vi "Dashboard Main.vi"() -> ()   [LabVIEW 2020]
uses:
  <vilib>/event_ctls.llb/eventvkey.ctl
  <vilib>/Rock Robotics/WPI/ThirdParty/JAS_Junk/TrajLib/TypeDef/TRANSLATION2D.ctl
  d5e2e769-f078-4149-bfe1-3f7844503895.vi
  <vilib>/Rock Robotics/WPI/ThirdParty/JAS_Junk/TrajLib/Conv_Radians_Deg.vi
  <vilib>/Rock Robotics/WPI/ThirdParty/JAS_Junk/TrajLib/Conv_Deg_Radians.vi
  <vilib>/Rock Robotics/WPI/ThirdParty/JAS_Junk/TrajLib/Rotation2d_CreateAngle.vi
  <vilib>/Rock Robotics/WPI/ThirdParty/JAS_Junk/TrajLib/Translation2d_Create.vi
  <vilib>/Rock Robotics/WPI/ThirdParty/JAS_Junk/TrajLib/VI/Util_GetTime_U32.vi
  <vilib>/Rock Robotics/Network Tables/NT Read Numeric Array.vi
  <vilib>/Rock Robotics/WPI/ThirdParty/JAS_Junk/TrajLib/VI/Util_GetTime_U64.vi
  <vilib>/Rock Robotics/WPI/Dashboard/WPI_DashboardLogging Global.vi
  <vilib>/picture/picture.llb/Draw True-Color Pixmap.vi
  <vilib>/Rock Robotics/WPI/ThirdParty/JAS_Junk/TrajLib/Trajectory_Library.lvlib
  <vilib>/vision/NI_Vision_Development_Module.lvlib
panel:
  in  "Camera Settings Right":T1={"Frame Rate"=30, "Compression"=30, "Size"=1, "DB Camera Config"=FALSE} {"Frame Rate" scale=1.0..30.0; "Compression" scale=100.0..-1.0; "Size" items=["640x480", "320x240", "160x120"]}
  in  "Camera Name Right":string(combo)="No Camera Selection"
  out "Camera Perf":string
  in  "Camera Settings":T1={"Frame Rate"=30, "Compression"=30, "Size"=1, "DB Camera Config"=FALSE} {"Frame Rate" scale=1.0..30.0; "Compression" scale=100.0..-1.0; "Size" items=["640x480", "320x240", "160x120"]}
  in  "TCP":refnum<k5>
  in  "Rec Mode":enum32{"Stop", "Record", "Playback"}(radio)
  out "Robot IP":string
  out "Image Message":string="Timeout in Camera Communications"
  in  "Dashboard Tab":T2(tab)
  in  "Select Auto":string(combo)="Select Autonomous ..."
  out "NT Connection":bool
  out "MotorChart R":cluster{"Numeric":dbl, "Numeric":dbl}(graph)
  out "MotorChart L":cluster{"Numeric":dbl, "Numeric":dbl}(graph)
  out "MotorSliders R":cluster{"MotorSlide1":dbl, "MotorSlide2":dbl} {"MotorSlide2" scale=-1.0..1.0 scale format="%#_2e"; "MotorSlide1" scale=-1.0..1.0 scale format="%#_2e"}
  out "MotorSliders L":cluster{"MotorSlide1":dbl, "MotorSlide2":dbl} {"MotorSlide2" scale=-1.0..1.0 scale format="%#_2e"; "MotorSlide1" scale=-1.0..1.0 scale format="%#_2e"}
  out "Gyro":dbl(knob) scale=0.0..360.0
  out "JS1 Z":dbl(slide) scale=-1.0..1.0 scale format="%#_2e"
  out "JS1 Graph":cluster{"X":dbl, "Y":dbl}[](graph)
  out "JS1 Buttons":T3
  out "JS2 Z":dbl(slide) scale=-1.0..1.0 scale format="%#_2e"
  out "JS2 Graph":cluster{"X":dbl, "Y":dbl}[](graph)
  out "JS2 Buttons":T3
  out "Mode":T4(ring)=enum."Auto Disabled"
  out "Right Camera Perf":cluster{"Bandwidth (Mbps)":dbl, "FPS":dbl}
  out "Camera Image Right":T5(plugin-control)
  in  "DB/String 9":string
  in  "DB/String 8":string
  in  "DB/String 7":string
  in  "DB/String 6":string
  in  "DB/String 5":string
  in  "DB/String 4":string
  in  "DB/String 3":string
  in  "DB/String 2":string
  in  "DB/String 1":string
  in  "DB/String 0":string
  in  "DB/Slider 0":dbl(slide) scale=0.0..5.0
  in  "DB/Slider 1":dbl(slide) scale=0.0..5.0
  in  "DB/Slider 2":dbl(slide) scale=0.0..5.0
  in  "DB/Slider 3":dbl(slide) scale=0.0..5.0
  out "DB/LED 3":bool
  out "DB/LED 2":bool
  out "DB/LED 1":bool
  out "DB/LED 0":bool
  in  "DB/Button 3":bool
  in  "DB/Button 2":bool
  in  "DB/Button 1":bool
  in  "DB/Button 0":bool caption="New Name"
  out "PID Chart":cluster{"X":dbl[], "Y":dbl[]}[](graph)
  out "LF PIDF":dbl[](array[numeric])
  out "c(t)":dbl
  out "time":dbl
  in  "PID Ctrl":dbl[](array[numeric])=[0.7, 0.0, 0.0]
  out "r(t)":dbl
  in  "PV (NT Name)":string="ActualPoseX"
  in  "SP (NT Name)":string="SamplePoseX"
  out "Field":cluster{dbl[], dbl[]}[](graph)
  out "Current Time":dbl
  in  "Test Slider":dbl(slide) scale=0.0..100.0 scale format="%#_3g"
  in  "On/Off":bool caption="Solenoid"
  in  "Test Name":u16(ring) items=["Select the test to run..."]
  in  "Test Tree":string(tree)
  in  "Motor":cluster{"Value":dbl, "Enable":bool} {"Value" scale=-1.0..1.0 scale format="%#_3g"}
  out "Progress":T6 {"Test Progress" scale=0.0..100.0}
  in  "Rev/Fwd":cluster{"Forward":bool, "Reverse":bool}
  in  "Test Ring":u16(ring) items=["Monochrome", "Color"]
  in  "CheckList":i32(listbox)
  out "Tree":string(tree)
  out "Camera Image":T5(plugin-control)
  out "Background":bool
  in  "Camera Name":string(combo)="No Camera Selection"
  # "HW"
  # "HW"
  # "Joysticks"
  # "Drive Motors"
  # "Front"
  # "Right"
  # "Left"
  # "Back"
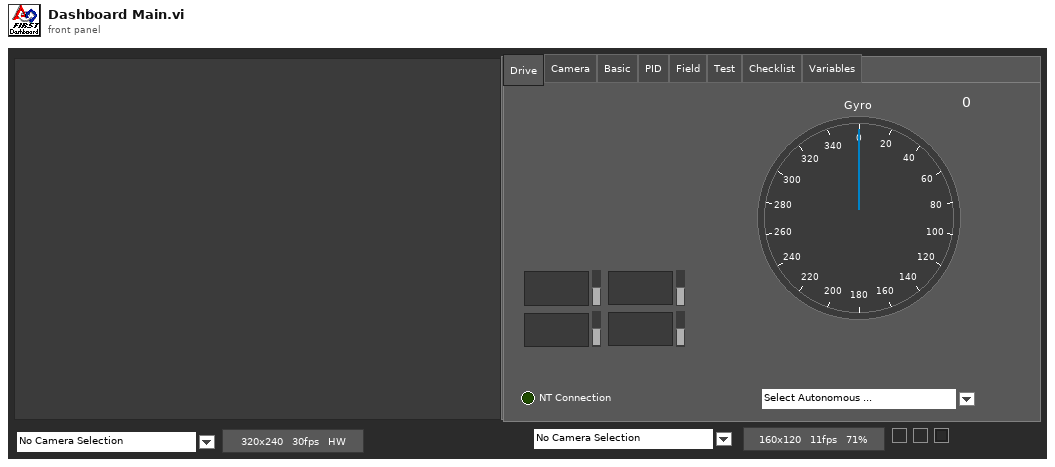
[diagram p1: front panel]
types:
  T1 = cluster{"Frame Rate":i32, "Compression":i32, "Size":u16, "DB Camera Config":bool}
  T2 = enum32{"Drive", "Camera", "Basic", "PID", "Field", "Test", "Checklist", "Variables"}
  T3 = cluster{bool, bool, bool, bool, bool, bool, bool, bool, bool, bool, bool, bool}
  T4 = enum8{"Tele-Op Disabled", "Tele-Op Enabled", "Auto Disabled", "Auto Enabled", "Test Disabled", "Test Enabled", "Disconnected", "No Code", "E-Stop"}
  T5 = typedef "IMAQ Image.ctl" = refnum<image>
  T6 = cluster{"Test Progress":u8, "Test Progress Text":string}
  T7 = typedef "Image Type" = u32
  T8 = cluster{"Save Path":path, "Interval (s)":dbl, "Keep":i32}
  T9 = enum32{"Drive", "Camera", "Basic", "Custom", "Test", "Commands", "Checklist", "Variables"}
  T10 = cluster{"Error Strings":string, "Disable Counts":cluster{u16, u16}, "Rail Faults":cluster{u16, u16, u16}, "Robot IP":string, "DB Mode":u8, "Event Info":cluster{"Name":string, "Type":u8, "Number":u16, "Replay":u8}}
  T11 = cluster{"Storage":cluster{"Disk Free":u64, "RAM Block":u32, "RAM free":u32}, "CPU Utilization":cluster{"CPU % ISR":sgl, "CPU % Time Crit":sgl, "CPU % Timed Str":sgl, "CPU % High":sgl, "CPU % Above":sgl, "CPU % Normal":sgl, "CPU % Low":sgl}, "CAN":cluster{"% Bus Utilization":sgl, "Bus Off Cnt":u32, "TX_FIFO Full Cnt":u32, "Receive Error Cnt":u8, "Transmit Error Cnt":u8}, "HID":cluster{"HID Outputs":u32, "Rumble Low":u16, "Rumble High":u16}[]}
  T12 = cluster{"Status bits":cluster{"Test Mode":bool, "Autonomous":bool, "Enabled":bool, "Code Start":bool, "Brownout":bool, "Reserved 2":bool, "Reserved 3":bool, "E-Stop":bool}, "Code Trace":cluster{"Disabled":bool, "TeleOp":bool, "Auto":bool, "Test":bool}, "Controller Type":enum16{"unknown", "cRIO", "roboRio"}, "Code?":enum16{"unknown", "noCode", "code"}, "Battery V":dbl}
  T13 = cluster{"Control Bits":cluster{"TestMode":bool, "Autonomous":bool, "Enabled":bool, "FMS Present":bool, bool, bool, bool, "E-Stop":bool}, "Team Station ":u8, "Countdown":sgl, "Joystick Values":cluster{"Axes":dbl[], "Buttons":bool[], "POVs":i16[]}[]}
  T14 = typedef "Trajectory_Library.lvlib/TRANSLATION2D.ctl" = cluster{"X":dbl, "Y":dbl}
  T15 = cluster{"Axes":dbl[], "Buttons":bool[], "POVs":i16[]}[]
  T16 = cluster{"Axes":dbl[], "Buttons":bool[], "POVs":i16[]}
  T17 = cluster{"Buttons[0]":bool, "Buttons[1]":bool, "Buttons[2]":bool, "Buttons[3]":bool, "Buttons[4]":bool, "Buttons[5]":bool, "Buttons[6]":bool, "Buttons[7]":bool, "Buttons[8]":bool, "Buttons[9]":bool, "Buttons[10]":bool, "Buttons[11]":bool}
  T18 = typedef "Trajectory_Library.lvlib/ROTATION2D.ctl" = cluster{"VALUE":dbl, "COS":dbl, "SIN":dbl}
  T19 = cluster{"Camera Image":refnum<vi>, "Dashboard Tab":refnum<vi>, "Background":refnum<vi>, "Rec Mode":refnum<vi>, "Test Slider":refnum<vi>, "On/Off ":refnum<vi>, "Test Ring":refnum<vi>, "Rev/Fwd":refnum<vi>, "Test Name":refnum<vi>, "Motor":refnum<vi>, "Progress":refnum<vi>, "CheckList":refnum<vi>, "Tree":refnum<vi>, "Test Tree":refnum<vi>, "Camera Settings":refnum<vi>, "Camera Name":refnum<vi>, "Camera Perf":refnum<vi>, "Camera Settings Right":refnum<vi>, "Camera Name Right":refnum<vi>, "Camera Image Right":refnum<vi>}
  T20 = cluster{"Global Rectangle":i32[], "Contours":cluster{"Contour Type":u32, "ROI Type":u32, "Points":i32[]}[]}
  T21 = cluster{"Camera Name":string, string, "Saved DB Images Info":cluster{"Save Path":path, "Interval (s)":dbl, "Keep":i32}}
  T22 = cluster{"Camera Name Right":string, string, "Saved DB Images Info":cluster{"Save Path":path, "Interval (s)":dbl, "Keep":i32}}
  T23 = cluster{"Operation":enum16{"Update", "Clear"}, "Color Box":u32}[]
  T24 = typedef "eventvkey.ctl" = enum16{"ASCII", "Enter", "Return", "Shift", "Ctrl", "Alt", "Cmd", "Opt", "Caps", "NumLock", "Clear", "Break", "Up", "Down", "Left", "Right", "Insert", "Delete", "Home", "End", "PageUp", "PageDown", "Escape", "Help", "Pause", "ScrollLock", "F1", "F2", "F3", "F4", "F5", "F6", "F7", "F8", "F9", "F10", "F11", "F12", "F13", "F14", "F15", "F16", "F17", "F18", "F19", "F20", "F21", "F22", "F23", "F24", "Play", "VolumeUp", "VolumeDown", "Mute", "Two Byte Char"}
  T25 = cluster{"Image Size":bool, "Image Type":bool, "Pixel Value":bool, "ROI Information":bool, "Zoom Factor":bool}
  T26 = cluster{"Operation":enum16{"Update", "Clear"}, "Color Box":u32}
  T27 = cluster{"Shift":bool, "Ctrl":bool, "Alt":bool, "Cmd":bool, "Opt":bool}
  T28 = typedef "imagedata.ctl" = cluster{"image type":i32, "image depth":i32, "image":u8[], "mask":u8[], "colors":u32[], "Rectangle":cluster{"left":i16, "top":i16, "right":i16, "bottom":i16}}
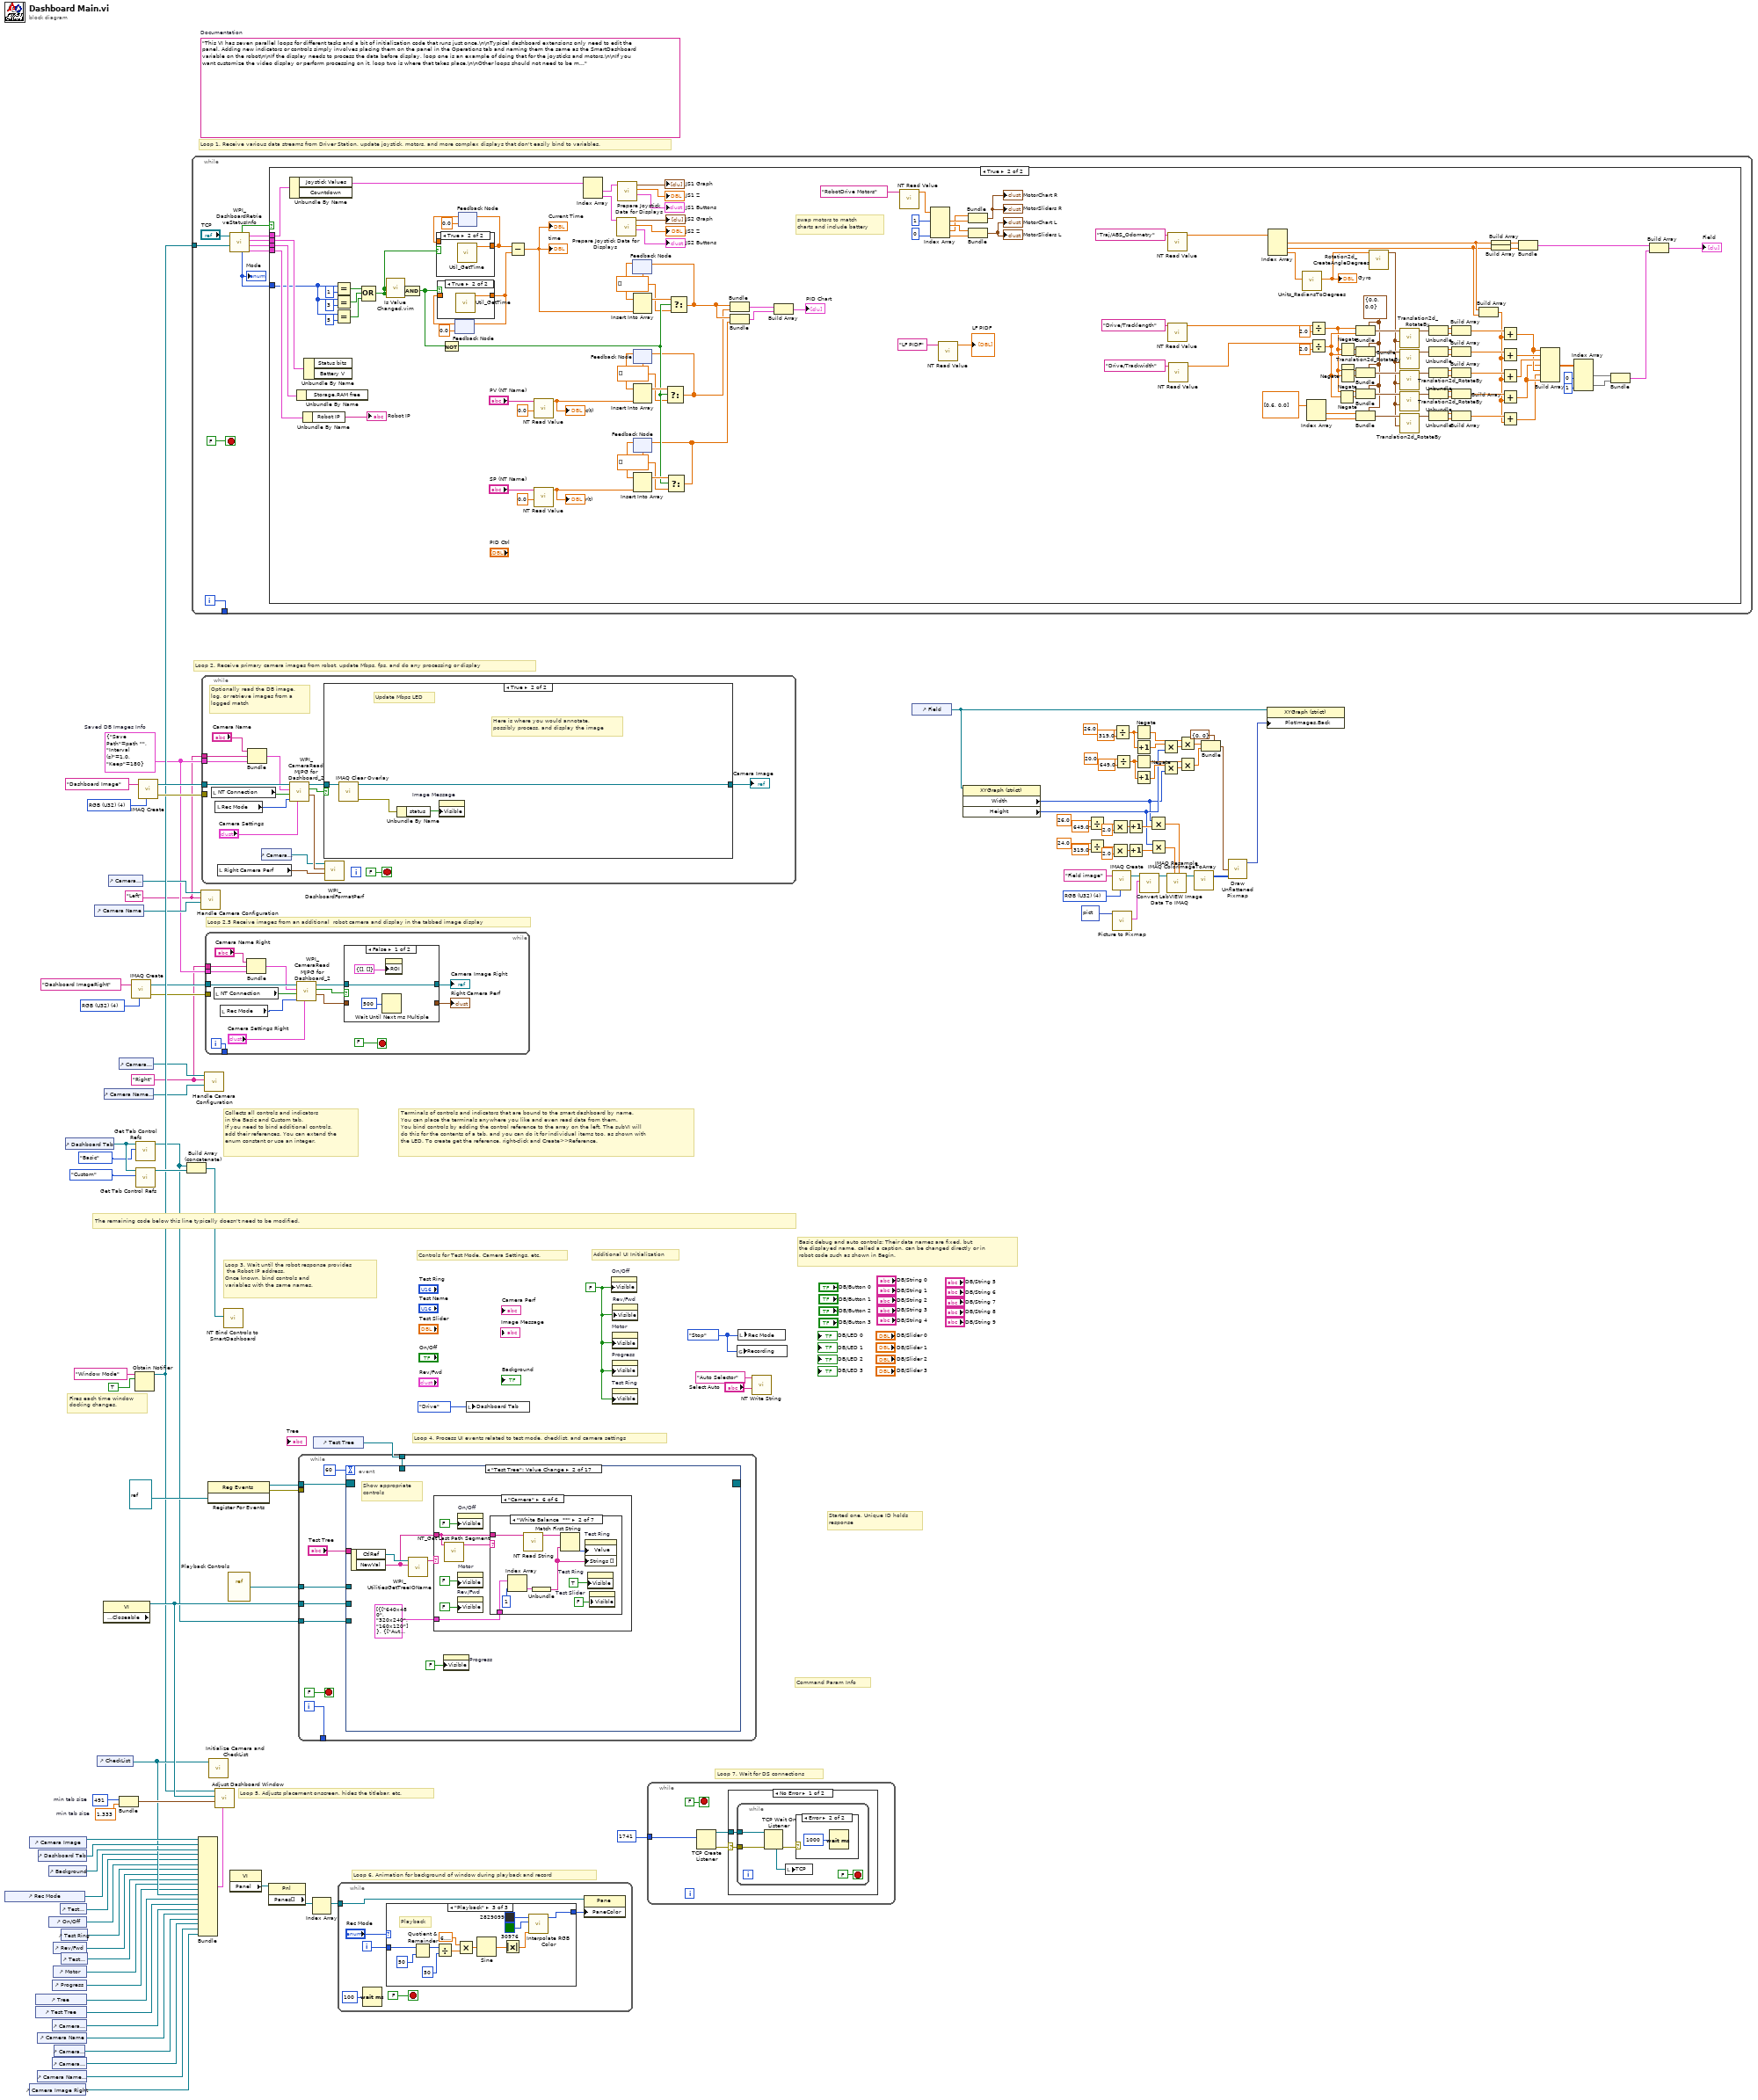
[diagram p0: block diagram]
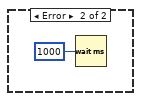
[diagram p4: hidden frame]
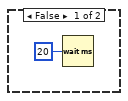
[diagram p5: hidden frame]
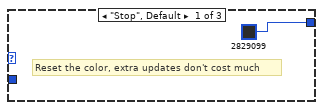
[diagram p8: hidden frame]
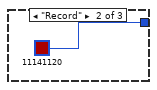
[diagram p9: hidden frame]
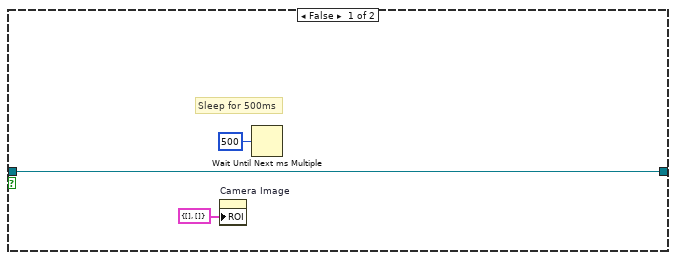
[diagram p10: hidden frame]
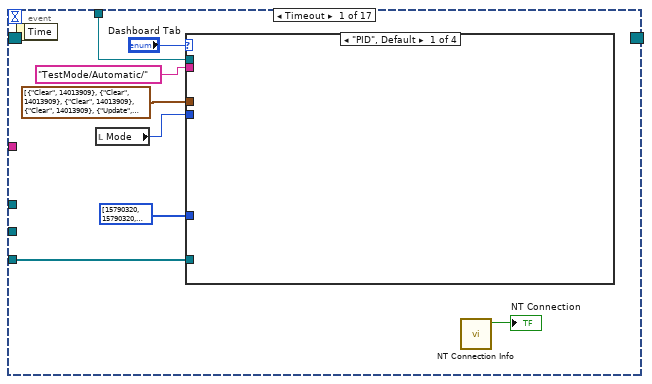
[diagram p11: hidden frame]
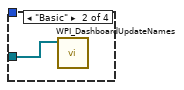
[diagram p12: hidden frame]
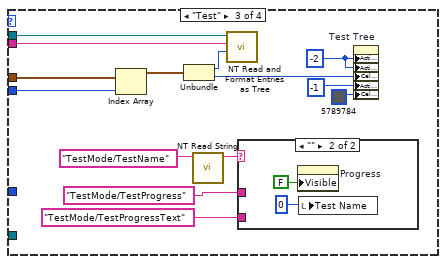
[diagram p13: hidden frame]
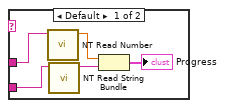
[diagram p14: hidden frame]
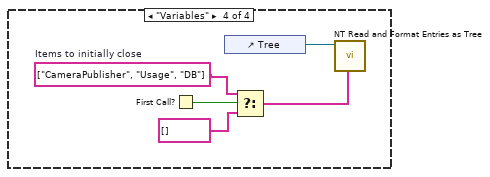
[diagram p15: hidden frame]
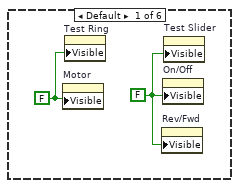
[diagram p16: hidden frame]
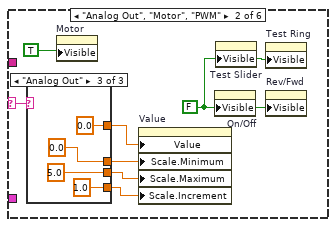
[diagram p17: hidden frame]
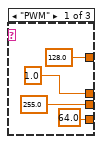
[diagram p18: hidden frame]
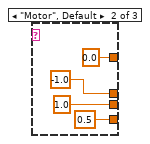
[diagram p19: hidden frame]
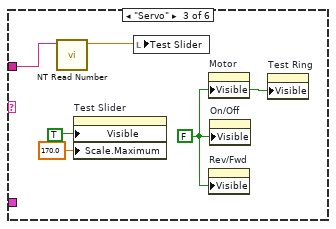
[diagram p20: hidden frame]
diagram:
  w40 = T7 4 items=["Grayscale (U8)", "Grayscale (I16)", "Grayscale (SGL)", "Complex (CSG)", "RGB (U32)", "HSL (U32)", "RGB (U64)", "Grayscale (U16)"] ("Image Type")
  w46 = T8 {"Save Path"=path "", "Interval (s)"=1.0, "Keep"=180}  # Saved DB Images Info
  w45 = "Right"
  w44 = "Left"
  w56 = T7 4 items=["Grayscale (U8)", "Grayscale (I16)", "Grayscale (SGL)", "Complex (CSG)", "RGB (U32)", "HSL (U32)", "RGB (U64)"] ("Image Type")
  w84 = 491  # min tab size
  w83 = 1.333  # min tab size
  w91 = enum32{"Stop", "Record", "Playback"}."Stop" ("Rec Mode")
  w68 = FALSE ("Visible")
  (unwired) "This VI has seven parallel loops for different tasks and a bit of initialization code that runs just once.\n\nTypical dashboard extensions only need to edit the panel. Adding new indicators or controls simply involves placing them on the panel in the Operations tab and naming them the same as the SmartDashboard variable on the robot\n\nIf the display needs to process the data before display, loop one is an example of doing that for the joysticks and motors.\n\nIf you want customize the video display or perform processing on it, loop two is where that takes place.\n\nOther loops should not need to be modified. They are pretty standard, and document the task they perform."  # Documentation
  w105 = T7 4 items=["Grayscale (U8)", "Grayscale (I16)", "Grayscale (SGL)", "Complex (CSG)", "RGB (U32)", "HSL (U32)", "RGB (U64)"] ("Image Type")
  # "Loop 2.5 Receive images from an additional  robot camera and display in the tabbed image display"
  # "Command Param Info"
  # "Started one, Unique ID holds\nresponse"
  # "Loop 7. Wait for DS connections"
  # "Basic debug and auto controls: Their data names are fixed, but\nthe displayed name, called a caption, can be changed directly or in\nrobot code such as shown in Begin."
  # "Controls for Test Mode, Camera Settings, etc."
  # "Additional UI Initialization"
  # "Loop 6. Animation for background of window during playback and record"
  # "Fires each time window\ndocking changes."
  # "Collects all controls and indicators\nin the Basic and Custom tab.\nIf you need to bind additional controls,\nadd their references. You can extend the\nenum constant or use an integer."
  # "The remaining code below this line typically doesn't need to be modified."
  # "Loop 4. Process UI events related to test mode, checklist, and camera settings"
  # "Terminals of controls and indicators that are bound to the smart dashboard by name.\nYou can place the terminals anywhere you like and even read data from them.\nYou bind controls by adding the control reference to the array on the left. The subVI will\ndo this for the contents of a tab, and you can do it for individual items too, as shown with\nthe LED. To create get the reference, right-click and Create>>Reference."
  # "Loop 3. Wait until the robot response provides\n the Robot IP address.\nOnce known, bind controls and\nvariables with the same names."
  # "Loop 5. Adjusts placement onscreen, hides the titlebar, etc."
  # "Loop 1. Receive various data streams from Driver Station, update joystick, motors, and more complex displays that don't easily bind to variables."
  # "Loop 2. Receive primary camera images from robot, update Mbps, fps, and do any processing or display"
  n1 = control-ref of="Rec Mode"() -> (w74:refnum<vi>)
  n2 = control-ref of="Camera Image Right"() -> (w49:refnum<vi>)
  n3 = control-ref of="Camera Image"() -> (w86:refnum<vi>)
  n4 = control-ref of="Tree"() -> (w78:refnum<vi>)
  n5 = control-ref of="Test Tree"() -> (w77:refnum<vi>)
  n6 = control-ref of="Camera Name"() -> (w62:refnum<vi>)
  n7 = control-ref of="Camera Name Right"() -> (w50:refnum<vi>)
  n8 = control-ref of="Dashboard Tab"() -> (w85:refnum<vi>)
  n9 = control-ref of="Background"() -> (w81:refnum<vi>)
  n10 = control-ref of="On/Off"() -> (w72:refnum<vi>)
  n11 = control-ref of="Progress"() -> (w69:refnum<vi>)
  n12 = control-ref of="Camera Settings"() -> (w63:refnum<vi>)
  n13 = control-ref of="Camera Settings Right"() -> (w51:refnum<vi>)
  n14 = control-ref of="Rev/Fwd"() -> (w70:refnum<vi>)
  n15 = control-ref of="Motor"() -> (w75:refnum<vi>)
  n16 = control-ref of="Camera Perf"() -> (w61:refnum<vi>)
  n17 = control-ref of="Test Slider"() -> (w73:refnum<vi>)
  n18 = control-ref of="Test Ring"() -> (w71:refnum<vi>)
  n19 = control-ref of="Test Name"() -> (w76:refnum<vi>)
  n20 = control-ref of="Dashboard Tab"() -> (w89:refnum<vi>)
  n21 = control-ref of="Camera Name"() -> (w64:refnum<vi>)
  n22 = control-ref of="CheckList"() -> (w79:refnum<vi>)
  n23 = property class="VI" props=["Front Panel.Closeable"]() -> (reference out=w90:refnum<vi>)  [unwired: 2 in, 2 out]
  n24 = control-ref of="Camera Name Right"() -> (w52:refnum<vi>)
  n25 = control-ref of="Camera Settings"() -> (w65:refnum<vi>)
  n26 = control-ref of="Camera Settings Right"() -> (w53:refnum<vi>)
  n27 = Bundle("min tab size"=w84, "min tab size"=w83) -> (w82:cluster{"min tab size":i32, "min tab size":dbl})  [unwired: 1 in]
  n28 = call "IMAQ Create"("Image Name"="Dashboard ImageRight", "Image Type"=w56) -> ("New Image"=w55:T5, "error out"=w54:errorcluster)  [unwired: 2 in, 1 out]
  n29 = Obtain Notifier(name (unnamed)="Window Mode", notification data type=TRUE) -> (notifier out=w67:refnum<notifier>)  [unwired: 2 in, 2 out]
  n30 = call <vilib>:"Get Tab Control Refs.vi"("Page Index"=T9."Basic" ("Dashboard Tab"), "TabControl in"=w89) -> ("ControlsOnPage"=w60:refnum<vi>[])  [unwired: 9 in]
  n31 = call <vilib>:"Get Tab Control Refs.vi"("Page Index"=T9."Custom" ("Dashboard Tab"), "TabControl in"=w89) -> ("ControlsOnPage"=w88:refnum<vi>[])  [unwired: 9 in]
  n32 = call "IMAQ Create"("Image Name"="Dashboard Image", "Image Type"=w105) -> ("New Image"=w103:T5, "error out"=w102:errorcluster)  [unwired: 2 in, 1 out]
  n33 = Build Array (concatenate)(w60, w88) -> (w87:refnum<vi>[])
  n34 = while {
    tunnel: [w114] -> _
    tunnel: w67 -> [w106]
    i -> [w114]
    stop <- FALSE stop-if-true
    n35 = call <vilib>:"WPI_DashboardRetrieveStatusInfo.vi"("Window Mode Notifier"=w106, "TCP Cnx"="TCP") -> ("Power and Errors"=w109:T10, "Robot Metrics"=w112:T11, "Status Info"=w113:T12, "Control Info"=w110:T13, "Robot Mode"=w108:T4, "Process?"=w111:bool)  [unwired: 4 in]
    "Mode" <- w108
    n36 = case shown="True" w111 {
      tunnel: w113 -> [_ w245]
      tunnel: w112 -> [_ w244]
      tunnel: w110 -> [_ w243]
      tunnel: w109 -> [_ w242]
      tunnel: w108 -> [_ w128]
      frame False {
        n37 = Wait (ms)(milliseconds to wait=u32 20) -> ()  [unwired: 1 out]
      }
      frame True {
        w123 = dbl[] []
        w153 = T14 {"X"=0.0, "Y"=0.0} ("In Translation")
        w122 = dbl[] []
        w121 = dbl[] []
        # "swap motors to match\ncharts and include battery"
        n38 = Unbundle By Name(w243) -> ("Joystick Values"=w233:T15)  [unwired: 1 out]
        n39 = Unbundle By Name(w244) -> ()  [unwired: 1 out]
        n40 = Unbundle By Name(w242) -> ("Robot IP"=→"Robot IP":string)
        n41 = Unbundle By Name(w245) -> ()  [unwired: 2 out]
        n42 = Equal?(x=w128, y=u32 1) -> (x = y?=w127:bool)
        n43 = Equal?(x=w128, y=u32 3) -> (x = y?=w126:bool)
        n44 = Equal?(x=w128, y=u32 5) -> (x = y?=w125:bool)
        n45 = Compound Arithmetic op=OR(w127, w126, w125) -> (w124:bool)
        n46 = call "Is Value Changed.vim"("value"=w124) -> ("changed or first call?"=w214:bool)
        n47 = And(x=w214, y=w124) -> (x .and. y?=w203:bool)
        n48 = Not(x=w203) -> (.not. x?=w133:bool)
        n49 = feedback #1(0.0 ("FPGA_Time_Seconds")) -> (w218:dbl)
        n50 = case shown="True" w203 {
          tunnel: [w248 w249] -> w217
          tunnel: w218 -> [w248 _]
          frame False {
          }
          frame True {
            n51 = call <vilib>:"Util_GetTime.vi"() -> ("FPGA_Time_Seconds"=w249:dbl)  [unwired: 9 in, 2 out]
          }
        }
        n52 = feedback-in #1(w217) -> ()
        n53 = feedback #2(0.0 ("FPGA_Time_Seconds")) -> (w208:dbl)
        n54 = case shown="True" w124 {
          tunnel: [w246 w247] -> w207
          tunnel: w208 -> [w246 _]
          frame False {
          }
          frame True {
            n55 = call <vilib>:"Util_GetTime.vi"() -> ("FPGA_Time_Seconds"=w247:dbl)  [unwired: 9 in, 2 out]
          }
        }
        n56 = feedback-in #2(w207) -> ()
        n57 = Subtract(x=w207, y=w217) -> (x-y=w201:dbl)
        "time" <- w201
        "Current Time" <- w201
        n58 = call-poly <vilib>:"NT Read Value.vi"("default value"=0.0, "name"="PV (NT Name)") -> ("value"=w211:dbl)  [unwired: 7 in, 2 out]
        "c(t)" <- w211
        n59 = call-poly <vilib>:"NT Read Value.vi"("default value"=0.0, "name"="SP (NT Name)") -> ("value"=w135:dbl)  [unwired: 7 in, 2 out]
        "r(t)" <- w135
        n60 = Index Array(array=w233) -> (element #1=w232:T16, element #2=w228:T16)  [unwired: 2 in]
        n61 = call "Prepare Joystick Data for Displays.vi"("Joystick Values"=w228) -> ("Buttons"=→"JS2 Buttons":T17, "Z Axis"=→"JS2 Z":dbl, "Cartesian Data"=→"JS2 Graph":cluster{"X axis":dbl, "X axis":dbl}[])  [unwired: 8 in]
        n62 = call "Prepare Joystick Data for Displays.vi"("Joystick Values"=w232) -> ("Buttons"=→"JS1 Buttons":T17, "Z Axis"=→"JS1 Z":dbl, "Cartesian Data"=→"JS1 Graph":cluster{"X axis":dbl, "X axis":dbl}[])  [unwired: 8 in]
        n63 = feedback #3(w121) -> (w213:dbl[])
        n64 = Insert Into Array(array=w213, new element=w201) -> (w205:dbl[])  [unwired: 1 in]
        n65 = feedback #4(w122) -> (w212:dbl[])
        n66 = Insert Into Array(array=w212, new element=w211) -> (w204:dbl[])  [unwired: 1 in]
        n67 = feedback #5(w123) -> (w136:dbl[])
        n68 = Insert Into Array(array=w136, new element=w135) -> (w134:dbl[])  [unwired: 1 in]
        n69 = Select(t=w204, s=w133, f=w122) -> (s? t:f=w119:dbl[])
        n70 = feedback-in #4(w119) -> ()
        n71 = Select(t=w134, s=w133, f=w123) -> (s? t:f=w132:dbl[])
        n72 = feedback-in #5(w132) -> ()
        n73 = Select(t=w205, s=w133, f=w121) -> (s? t:f=w120:dbl[])
        n74 = feedback-in #3(w120) -> ()
        n75 = Bundle(w120, w119) -> (w210:cluster{dbl[], dbl[]})  [unwired: 1 in]
        n76 = Bundle(w120, w132) -> (w131:cluster{dbl[], dbl[]})  [unwired: 1 in]
        n77 = Build Array(w210, w131) -> (→"PID Chart":cluster{dbl[], dbl[]}[])
        n78 = call-poly <vilib>:"NT Read Value.vi"("name"="RobotDrive Motors" ("Name")) -> ("value"=w223:dbl[])  [unwired: 8 in, 2 out]
        n79 = Index Array(array=w223, index #1=1, index #4=0) -> (element #1=w237:dbl, element #2=w238:dbl, element #3=w236:dbl, element #4=w241:dbl)  [unwired: 2 in]
        n80 = call-poly <vilib>:"NT Read Value.vi"("name"="LF PIDF") -> ("value"=→"LF PIDF":dbl[])  [unwired: 8 in, 2 out]
        n81 = Bundle("Numeric"=w236, "Numeric"=w237) -> (→"MotorChart R" →"MotorSliders R":cluster{"Numeric":dbl, "Numeric":dbl})  [unwired: 1 in]
        n82 = Bundle("Numeric"=w238, "Numeric"=w241) -> (→"MotorChart L" →"MotorSliders L":cluster{"Numeric":dbl, "Numeric":dbl})  [unwired: 1 in]
        n83 = call-poly <vilib>:"NT Read Value.vi"("name"="Traj/ABS_Odometry") -> ("value"=w151:dbl[])  [unwired: 8 in, 2 out]
        n84 = call-poly <vilib>:"NT Read Value.vi"("name"="Drive/Tracklength" ("Name")) -> ("value"=w141:dbl)  [unwired: 8 in, 2 out]
        n85 = call-poly <vilib>:"NT Read Value.vi"("name"="Drive/Trackwidth" ("Name")) -> ("value"=w140:dbl)  [unwired: 8 in, 2 out]
        n86 = Index Array(array=w151) -> (element #1=w150:dbl, element #2=w149:dbl, element #3=w139:dbl)  [unwired: 3 in]
        n87 = call <vilib>:"Units_RadiansToDegrees.vi"("Radians"=w139) -> ("Degrees"=w138:dbl)  [unwired: 10 in]
        "Gyro" <- w138
        n88 = Index Array(array=dbl[] [0.6, 0.0] ("y")) -> (element #1=w155:dbl, element #2=w154:dbl)  [unwired: 2 in]
        n89 = Divide(x=w141, y=2.0) -> (x/y=w186:dbl)
        n90 = Divide(x=w140, y=2.0) -> (x/y=w187:dbl)
        n91 = Negate(x=w187) -> (-x=w162:dbl)
        n92 = Negate(x=w186) -> (-x=w190:dbl)
        n93 = Negate(x=w186) -> (-x=w189:dbl)
        n94 = Negate(x=w187) -> (-x=w188:dbl)
        n95 = Bundle(cluster=w153, "X"=w186, "Y"=w187) -> (w198:T14)
        n96 = Bundle(cluster=w153, "X"=w190, "Y"=w187) -> (w194:T14)
        n97 = Bundle(cluster=w153, "X"=w189, "Y"=w188) -> (w193:T14)
        n98 = Bundle(cluster=w153, "X"=w186, "Y"=w162) -> (w192:T14)
        n99 = Bundle(cluster=w153, "X"=w155, "Y"=w154) -> (w163:T14)
        n100 = call <vilib>:"Rotation2d_CreateAngleDegrees.vi"("Angle_Degrees"=w138) -> ("ROTATION"=w161:T18)  [unwired: 10 in]
        n101 = call <vilib>:"Translation2d_RotateBy.vi"("other Rotation"=w161, "In Translation"=w198) -> ("Out Translation"=w197:T14)  [unwired: 9 in]
        n102 = call <vilib>:"Translation2d_RotateBy.vi"("other Rotation"=w161, "In Translation"=w194) -> ("Out Translation"=w196:T14)  [unwired: 9 in]
        n103 = call <vilib>:"Translation2d_RotateBy.vi"("other Rotation"=w161, "In Translation"=w193) -> ("Out Translation"=w195:T14)  [unwired: 9 in]
        n104 = call <vilib>:"Translation2d_RotateBy.vi"("other Rotation"=w161, "In Translation"=w192) -> ("Out Translation"=w191:T14)  [unwired: 9 in]
        n105 = call <vilib>:"Translation2d_RotateBy.vi"("other Rotation"=w161, "In Translation"=w163) -> ("Out Translation"=w164:T14)  [unwired: 9 in]
        n106 = Unbundle(w197) -> ("X"=w185:dbl, "Y"=w184:dbl)
        n107 = Unbundle(w196) -> ("X"=w182:dbl, "Y"=w183:dbl)
        n108 = Unbundle(w195) -> ("X"=w181:dbl, "Y"=w180:dbl)
        n109 = Unbundle(w191) -> ("X"=w179:dbl, "Y"=w178:dbl)
        n110 = Unbundle(w164) -> ("X"=w160:dbl, "Y"=w165:dbl)
        n111 = Build Array(w185, w184) -> (w177:dbl[])
        n112 = Build Array(w182, w183) -> (w176:dbl[])
        n113 = Build Array(w181, w180) -> (w175:dbl[])
        n114 = Build Array(w179, w178) -> (w174:dbl[])
        n115 = Build Array(w160, w165) -> (w158:dbl[])
        n116 = Build Array(w150, w149) -> (w152:dbl[])
        n117 = Build Array(w150) -> (w148:dbl[])
        n118 = Build Array(w149) -> (w147:dbl[])
        n119 = Add(x=w177, y=w152) -> (x+y=w171:dbl[])
        n120 = Add(x=w176, y=w152) -> (x+y=w173:dbl[])
        n121 = Add(x=w175, y=w152) -> (x+y=w172:dbl[])
        n122 = Add(x=w174, y=w152) -> (x+y=w159:dbl[])
        n123 = Add(x=w158, y=w152) -> (x+y=w157:dbl[])
        n124 = Bundle(w148, w147) -> (w146:cluster{dbl[], dbl[]})  [unwired: 1 in]
        n125 = Build Array(w171, w173, w172, w159, w171, w157, w159) -> (w170:dbl[][])
        n126 = Index Array(array=w170, index (col) #1=0 ("disabled index (col)"), index (col) #2=1 ("index (col)")) -> (element #1=w168:dbl[], element #2=w166:dbl[])  [unwired: 2 in]
        n127 = Bundle(w168, w166) -> (w145:cluster{dbl[], dbl[]})  [unwired: 1 in]
        n128 = Build Array(w146, w145) -> (→"Field":cluster{dbl[], dbl[]}[])
      }
    }
  }
  n129 = Bundle("Camera Image"=w86, "Dashboard Tab"=w85, "Background"=w81, "Rec Mode"=w74, "Test Slider"=w73, "On/Off"=w72, "Test Ring"=w71, "Rev/Fwd"=w70, "Test Name"=w76, "Motor"=w75, "Progress"=w69, "CheckList"=w79, "Tree"=w78, "Test Tree"=w77, "Camera Settings"=w63, "Camera Name"=w62, "Camera Perf"=w61, "Camera Settings Right"=w51, "Camera Name Right"=w50, "Camera Image Right"=w49) -> (w80:T19)  [unwired: 1 in]
  n130 = call "Handle Camera Configuration.vi"("CameraNameRef"=w64, "Display Name"=w44, "ClusterRef"=w65) -> ()  [unwired: 9 in]
  n131 = while {
    tunnel: w103 -> [w263]
    tunnel: w102 -> [_]
    tunnel: w46 -> [w256]
    tunnel: w44 -> [w253]
    stop <- FALSE stop-if-true
    # "Optionally read the DB image,\nlog, or retrieve images from a\nlogged match"
    n132 = local read "NT Connection"() -> (w257:bool)
    n133 = local read "Rec Mode"() -> (w260:enum32{"Stop", "Record", "Playback"})
    n134 = local read "Right Camera Perf"() -> (w251:cluster{"Bandwidth (Mbps)":dbl, "FPS":dbl})
    n135 = Bundle("Camera Name"="Camera Name", w253, "Saved DB Images Info"=w256) -> (w255:T21)  [unwired: 1 in]
    n136 = control-ref of="Camera Perf"() -> (w250:refnum<vi>)
    n137 = call <vilib>:"WPI_CameraRead MJPG for Dashboard_2.vi"("Camera Settings"="Camera Settings", "Rec Mode"=w260, "NT Connection"=w257, "Capture Info"=w255, "Image in"=w263) -> ("perf info"=w252:cluster{"Bandwidth (Mbps)":dbl, "fps":dbl}, "Active"=w261:bool, "Image\\ out"=w262:T5)  [unwired: 4 in]
    n138 = case shown="True" w261 {
      tunnel: w262 -> [w266 w269]
      tunnel: [w266 w268] -> w258
      frame False {
        # "Sleep for 500ms"
        n139 = property on="Camera Image" class="ImageControl"("ROI"=T20 {"Global Rectangle"=[], "Contours"=[]}) -> ()  [unwired: 2 in, 2 out]
        n140 = Wait Until Next ms Multiple(millisecond multiple=u32 500) -> ()  [unwired: 1 out]
      }
      frame True {
        # "Here is where you would annotate,\npossibly process, and display the image"
        # "Update Mbps LED"
        n141 = call "IMAQ Clear Overlay"("Image"=w269) -> ("error out"=w270:errorcluster, "Image Out"=w268:T5)  [unwired: 2 in, 7 out]
        n142 = Unbundle By Name(w270) -> ("status"=w271:bool)
        n143 = property on="Image Message" class="Str"("Visible"=w271) -> ()  [unwired: 2 in, 2 out]
      }
    }
    "Camera Image" <- w258
    n144 = call <vilib>:"WPI_DashboardFormatPerf.vi"("Right Camera Perf"=w251, "Performance"=w252, "String in"=w250) -> ()  [unwired: 9 in]
  }
  n145 = call "Handle Camera Configuration.vi"("CameraNameRef"=w52, "Display Name"=w45, "ClusterRef"=w53) -> ()  [unwired: 9 in]
  n146 = while {
    tunnel: w55 -> [w286]
    tunnel: w54 -> [_]
    tunnel: [w281] -> _
    tunnel: w46 -> [w277]
    tunnel: w45 -> [w274]
    i -> [w281]
    stop <- FALSE stop-if-true
    n147 = local read "NT Connection"() -> (w278:bool)
    n148 = local read "Rec Mode"() -> (w285:enum32{"Stop", "Record", "Playback"})
    n149 = Bundle("Camera Name Right"="Camera Name Right", w274, "Saved DB Images Info"=w277) -> (w276:T22)  [unwired: 1 in]
    n150 = call <vilib>:"WPI_CameraRead MJPG for Dashboard_2.vi"("Camera Settings"="Camera Settings Right", "Rec Mode"=w285, "NT Connection"=w278, "Capture Info"=w276, "Image in"=w286) -> ("perf info"=w272:cluster{"Bandwidth (Mbps)":dbl, "fps":dbl}, "Active"=w280:bool, "Image\\ out"=w283:T5)  [unwired: 4 in]
    n151 = case shown="False" w280 {
      tunnel: w283 -> [w288 w291]
      tunnel: [w288 w291] -> w279
      tunnel: [_ w290] -> w273
      tunnel: w272 -> [_ w290]
      frame False {
        n152 = Wait Until Next ms Multiple(millisecond multiple=u32 500) -> ()  [unwired: 1 out]
        n153 = property on="Camera Image Right" class="ImageControl"("ROI"=T20 {"Global Rectangle"=[], "Contours"=[]}) -> ()  [unwired: 2 in, 2 out]
      }
      frame True {
      }
    }
    "Camera Image Right" <- w279
    "Right Camera Perf" <- w273
  }
  n154 = register-events(refnum<vi> refnum) -> (reference out=w94:refnum<event-registration>, error out=w93:errorcluster)  [unwired: 2 in]
  n155 = call "Initialize Camera and CheckList.vi"("ListBox in"=w79) -> ()  [unwired: 11 in]
  n156 = call "Adjust Dashboard Window.vi"("Sizing Refnums"=w80, "Size Constraints"=w82, "VI"=w90, "WIn Mode"=w67) -> ()  [unwired: 8 in]
  n157 = call <vilib>:"NT Bind Controls to SmartDashboard.vi"("Bound Control Refs"=w87) -> ()  [unwired: 11 in]
  n158 = vi-ref "Playback Controls.vi"() -> (w95:refnum<vi>)
  n159 = property class="VI"() -> ("Panel"=w97:refnum<vi>)  [unwired: 2 in, 2 out]
  n160 = property class="Pnl"(reference=w97) -> ("Panes[]"=w98:refnum<vi>[])  [unwired: 1 in, 2 out]
  n161 = Index Array(array=w98) -> (element=w96:refnum<vi>)  [unwired: 1 in]
  n162 = control-ref of="Test Tree"() -> (w99:refnum<vi>)
  n163 = while {
    tunnel: [w297] -> _
    tunnel: w99 -> [w296]
    tunnel: w95 -> [w295]
    tunnel: w94 -> [w294]
    tunnel: w93 -> [_]
    tunnel: w90 -> [w293]
    tunnel: w60 -> [w292]
    i -> [w297]
    stop <- FALSE stop-if-true
    n164 = event shown="[1] \"Test Tree\": Value Change" {
      selector: w294 -> [_ _ _ _ _ _ _ _ _ _ _ _ _ _ _ _ _]
      dyn-events: [_ _ _ _ _ _ _ _ _ _ _ _ _ w502 _ _ _] -> _
      timeout: u32 60 ("milliseconds to wait") -> [_ _ _ _ _ _ _ _ _ _ _ _ _ _ _ _ _]
      tunnel: w296 -> [w307 _ _ _ _ _ _ _ _ _ _ _ _ _ _ _ _]
      tunnel: "Test Tree" -> [_ _ _ _ _ _ _ _ w475 w482 w483 w486 w493 _ _ _ _]
      tunnel: w295 -> [_ _ _ _ _ _ _ _ _ _ _ _ _ w504 _ w519 _]
      tunnel: w293 -> [_ _ _ _ _ _ _ _ _ _ _ _ _ w500 _ _ _]
      tunnel: w292 -> [w302 _ _ _ _ _ _ _ _ _ _ _ _ _ _ _ _]
      event Timeout {
        n165 = event-data() -> ()  [unwired: 1 in, 1 out]
        n166 = local read "Mode"() -> (w305:T4)
        n167 = case shown="\"PID\", Default" "Dashboard Tab" {
          tunnel: w307 -> [_ _ w323 _]
          tunnel: "TestMode/Automatic/" ("Name Pattern") -> [_ _ w322 _]
          tunnel: T23 [{"Operation"=enum."Clear", "Color Box"=14013909}, {"Operation"=enum."Clear", "Color Box"=14013909}, {"Operation"=enum."Clear", "Color Box"=14013909}, {"Operation"=enum."Clear", "Color Box"=14013909}, {"Operation"=enum."Update", "Color Box"=14013909}, {"Operation"=enum."Update", "Color Box"=16777215}, {"Operation"=enum."Clear", "Color Box"=14013909}, {"Operation"=enum."Clear", "Color Box"=14013909}, {"Operation"=enum."Clear", "Color Box"=14013909}] -> [_ _ w315 _]
          tunnel: w305 -> [_ _ w314 _]
          tunnel: u32[] [15790320, 15790320, 15790320, 15790320, 16777215, 16777215, 15790320, 15790320, 15790320] -> [_ _ _ _]
          tunnel: w302 -> [_ w309 _ _]
          frame "PID", Default {
          }
          frame "Basic" {
            n168 = call <vilib>:"WPI_DashboardUpdateNames.vi"("Controls on Tab"=w309) -> ()  [unwired: 11 in]
          }
          frame "Test" {
            w321 = -2 ("Active Item:Row Number")
            n169 = Index Array(array=w315, index=w314) -> (element=w316:T26)
            n170 = Unbundle(w316) -> ("Operation"=w317:enum16{"Update", "Clear"}, "Color Box"=w318:u32)
            n171 = call <vilib>:"NT Read String.vi"("name"="TestMode/TestName" ("Name")) -> ("value"=w312:string)  [unwired: 8 in, 2 out]
            n172 = call <vilib>:"NT Read and Format Entries as Tree.vi"("Operation"=w317, "Name Pattern"=w322, "Tree Refnum"=w323) -> ()  [unwired: 7 in, 2 out]
            n173 = case shown="\"\"" w312 {
              tunnel: "TestMode/TestProgress" ("Name") -> [w325 _]
              tunnel: "TestMode/TestProgressText" ("Name") -> [w324 _]
              frame Default {
                n174 = call <vilib>:"NT Read Number.vi"("name"=w325) -> ("value"=w326:dbl)  [unwired: 8 in, 2 out]
                n175 = call <vilib>:"NT Read String.vi"("name"=w324) -> ("value"=w327:string)  [unwired: 8 in, 2 out]
                n176 = Bundle("value"=w326, "value"=w327) -> (→"Progress":cluster{"value":dbl, "value":string})  [unwired: 1 in]
              }
              frame "" {
                n177 = property on="Progress" class="Clust (strict)"("Visible"=FALSE) -> ()  [unwired: 2 in, 2 out]
                n178 = local write "Test Name"(u16 0) -> ()
              }
            }
            n179 = property on="Test Tree" class="Tree (strict)"("Active Item Row Number"=w321, "ActiveColNum"=w321, "CellBG"=w318, "Active Item Row Number"=-1 ("Active Item:Row Number"), "CellBG"=u32 5789784 ("Color Box")) -> ()  [unwired: 2 in, 2 out]
          }
          frame "Variables" {
            w333 = string[] ["CameraPublisher", "Usage", "DB"]  # Items to initially close
            n180 = First Call?() -> (First Call?: T/F=w334:bool)
            n181 = control-ref of="Tree"() -> (w335:refnum<vi>)
            n182 = Select(t=w333, s=w334, f=string[] []) -> (s? t:f=w331:string[])
            n183 = call <vilib>:"NT Read and Format Entries as Tree.vi"("Tags to  Close"=w331, "Tree Refnum"=w335) -> ()  [unwired: 8 in, 2 out]
          }
        }
        n184 = call <vilib>:"NT Connection Info.vi"() -> ("Connected"=→"NT Connection":bool)  [unwired: 11 in]
      }
      event "Test Tree": Value Change {
        # "Show appropriate\ncontrols"
        n185 = event-data() -> ("CtlRef"=w339:refnum<vi>, "NewVal"=w337:string)  [unwired: 1 in]
        n186 = call <vilib>:"WPI_UtilitiesGetTreeIOName.vi"("NewVal"=w337, "TreeControl in"=w339) -> ("I/O Name"=w340:string)  [unwired: 9 in]
        n187 = case shown="\"Camera\"" w340 {
          selector: w340 -> [_ w347 _ w369 w378 _]
          tunnel: w337 -> [_ _ w366 w368 _ w385]
          tunnel: cluster{string[]}[] [{["640x480", "320x240", "160x120"]}, {["Auto", "Fixed indoor", "Fixed outdoor 1", "Fixed outdoor 2", "Fixed fluorescent 1", "Fixed fluorescent 2", "Hold current"]}, {["Auto", "Flicker-free 50 Hz", "Flicker-free 60 Hz", "Hold current"]}, {["None", "Prioritize frame rate", "Prioritize image quality"]}, {["Monochrome", "Color"]}] -> [_ _ _ _ _ w384]
          frame Default {
            w342 = FALSE ("Visible")
            w341 = FALSE ("Visible")
            n188 = property on="Motor" class="Clust (strict)"("Visible"=w341) -> ()  [unwired: 2 in, 2 out]
            n189 = property on="Test Ring" class="Ring (strict)"("Visible"=w341) -> ()  [unwired: 2 in, 2 out]
            n190 = property on="Rev/Fwd" class="Clust (strict)"("Visible"=w342) -> ()  [unwired: 2 in, 2 out]
            n191 = property on="On/Off" class="Bool (strict)"("Visible"=w342) -> ()  [unwired: 2 in, 2 out]
            n192 = property on="Test Slider" class="Slide (strict)"("Visible"=w342) -> ()  [unwired: 2 in, 2 out]
          }
          frame "Analog Out", "Motor", "PWM" {
            w348 = FALSE ("Visible")
            n193 = case shown="\"Analog Out\"" w347 {
              tunnel: [1.0 ("Value") -1.0 ("Value") 0.0 ("Value")] -> w346
              tunnel: [255.0 ("Value") 1.0 ("Value") 5.0 ("Value")] -> w345
              tunnel: [128.0 ("Value") 0.0 ("Value") 0.0 ("Value")] -> w344
              tunnel: [64.0 ("Value") 0.5 ("Value") 1.0 ("Value")] -> w343
              frame "PWM" {
              }
              frame "Motor", Default {
              }
              frame "Analog Out" {
              }
            }
            n194 = property on="Motor" class="Clust (strict)"("Visible"=TRUE) -> ()  [unwired: 2 in, 2 out]
            n195 = property on="Value" class="Slide (strict)"("Value"=w344, "Scale.Minimum"=w346, "Scale.Maximum"=w345, "Scale.Increment"=w343) -> ()  [unwired: 2 in, 2 out]
            n196 = property on="On/Off" class="Bool (strict)"("Visible"=w348) -> ()  [unwired: 2 in, 2 out]
            n197 = property on="Test Slider" class="Slide (strict)"("Visible"=w348) -> ()  [unwired: 2 in, 2 out]
            n198 = property on="Test Ring" class="Ring (strict)"("Visible"=w348) -> ()  [unwired: 2 in, 2 out]
            n199 = property on="Rev/Fwd" class="Clust (strict)"("Visible"=w348) -> ()  [unwired: 2 in, 2 out]
          }
          frame "Servo" {
            w364 = FALSE ("Visible")
            n200 = call <vilib>:"NT Read Number.vi"("name"=w366) -> ("value"=w365:dbl)  [unwired: 8 in, 2 out]
            n201 = property on="Test Slider" class="Slide (strict)"("Visible"=TRUE, "Scale.Maximum"=170.0 ("Scale.Range:Maximum")) -> ()  [unwired: 2 in, 2 out]
            n202 = local write "Test Slider"(w365) -> ()
            n203 = property on="Motor" class="Clust (strict)"("Visible"=w364) -> ()  [unwired: 2 in, 2 out]
            n204 = property on="Rev/Fwd" class="Clust (strict)"("Visible"=w364) -> ()  [unwired: 2 in, 2 out]
            n205 = property on="On/Off" class="Bool (strict)"("Visible"=w364) -> ()  [unwired: 2 in, 2 out]
            n206 = property on="Test Ring" class="Ring (strict)"("Visible"=w364) -> ()  [unwired: 2 in, 2 out]
          }
          frame "Relay", "Solenoid" {
            w367 = FALSE ("Visible")
            n207 = property on="Motor" class="Clust (strict)"("Visible"=w367) -> ()  [unwired: 2 in, 2 out]
            n208 = property on="Test Slider" class="Slide (strict)"("Visible"=w367) -> ()  [unwired: 2 in, 2 out]
            n209 = Search and Replace String(input string=w368, search string="/Value  **", replace string="/Direction") -> (result string=w374:string)  [unwired: 5 in, 3 out]
            n210 = property on="Test Ring" class="Ring (strict)"("Visible"=w367) -> ()  [unwired: 2 in, 2 out]
            n211 = call <vilib>:"NT Read String.vi"("name"=w374) -> ("value"=w372:string)  [unwired: 8 in, 2 out]
            n212 = Equal?(x="Both directions", y=w372) -> (x = y?=w370:bool)
            n213 = Not(x=w370) -> (.not. x?=w371:bool)
            n214 = property on="Rev/Fwd" class="Clust (strict)"("Visible"=w370) -> ()  [unwired: 2 in, 2 out]
            n215 = property on="On/Off" class="Bool (strict)"("Visible"=w371, "Caption.Text"=w369) -> ()  [unwired: 2 in, 2 out]
          }
          frame "Compressor", "Digital Out" {
            w377 = FALSE ("Visible")
            # "Get direction and finish"
            n216 = property on="Motor" class="Clust (strict)"("Visible"=w377) -> ()  [unwired: 2 in, 2 out]
            n217 = property on="Test Slider" class="Slide (strict)"("Visible"=w377) -> ()  [unwired: 2 in, 2 out]
            n218 = property on="Test Ring" class="Ring (strict)"("Visible"=w377) -> ()  [unwired: 2 in, 2 out]
            n219 = property on="On/Off" class="Bool (strict)"("Visible"=TRUE, "Caption.Text"=w378) -> ()  [unwired: 2 in, 2 out]
            n220 = property on="Rev/Fwd" class="Clust (strict)"("Visible"=FALSE) -> ()  [unwired: 2 in, 2 out]
          }
          frame "Camera" {
            n221 = call <vilib>:"NT_Get Last Path Segment.vi"("String in"=w385) -> ("String out"=w386:string)  [unwired: 10 in]
            n222 = property on="On/Off" class="Bool (strict)"("Visible"=FALSE) -> ()  [unwired: 2 in, 2 out]
            n223 = property on="Motor" class="Clust (strict)"("Visible"=FALSE) -> ()  [unwired: 2 in, 2 out]
            n224 = property on="Rev/Fwd" class="Clust (strict)"("Visible"=FALSE) -> ()  [unwired: 2 in, 2 out]
            n225 = case shown="\"White Balance  **\"" w386 {
              tunnel: w385 -> [w392 w401 w410 w419 w428 _ w434]
              tunnel: w384 -> [w390 w398 w407 w416 w425 _ _]
              frame "Size  **" {
                n226 = Index Array(array=w390) -> (element=w389:cluster{string[]})  [unwired: 1 in]
                n227 = call <vilib>:"NT Read String.vi"("name"=w392) -> ("value"=w391:string)  [unwired: 8 in, 2 out]
                n228 = Unbundle(w389) -> (w387:string[])
                n229 = Match First String(2:w387, 3:w391) -> (0:w388:i32)  [unwired: 1 out]
                n230 = property on="Test Ring" class="Ring (strict)"("Value"=w388, "Strings []"=w387) -> ()  [unwired: 2 in, 2 out]
                n231 = property on="Test Ring" class="Ring (strict)"("Visible"=TRUE) -> ()  [unwired: 2 in, 2 out]
                n232 = property on="Test Slider" class="Slide (strict)"("Visible"=FALSE) -> ()  [unwired: 2 in, 2 out]
              }
              frame "White Balance  **" {
                n233 = Index Array(array=w398, index=1) -> (element=w399:cluster{string[]})
                n234 = call <vilib>:"NT Read String.vi"("name"=w401) -> ("value"=w400:string)  [unwired: 8 in, 2 out]
                n235 = Unbundle(w399) -> (w396:string[])
                n236 = Match First String(2:w396, 3:w400) -> (0:w395:i32)  [unwired: 1 out]
                n237 = property on="Test Ring" class="Ring (strict)"("Value"=w395, "Strings []"=w396) -> ()  [unwired: 2 in, 2 out]
                n238 = property on="Test Ring" class="Ring (strict)"("Visible"=TRUE) -> ()  [unwired: 2 in, 2 out]
                n239 = property on="Test Slider" class="Slide (strict)"("Visible"=FALSE) -> ()  [unwired: 2 in, 2 out]
              }
              frame "Exposure  **" {
                n240 = Index Array(array=w407, index=2) -> (element=w408:cluster{string[]})
                n241 = call <vilib>:"NT Read String.vi"("name"=w410) -> ("value"=w409:string)  [unwired: 8 in, 2 out]
                n242 = Unbundle(w408) -> (w404:string[])
                n243 = Match First String(2:w404, 3:w409) -> (0:w405:i32)  [unwired: 1 out]
                n244 = property on="Test Ring" class="Ring (strict)"("Value"=w405, "Strings []"=w404) -> ()  [unwired: 2 in, 2 out]
                n245 = property on="Test Ring" class="Ring (strict)"("Visible"=TRUE) -> ()  [unwired: 2 in, 2 out]
                n246 = property on="Test Slider" class="Slide (strict)"("Visible"=FALSE) -> ()  [unwired: 2 in, 2 out]
              }
              frame "Exposure Priority  **" {
                n247 = Index Array(array=w416, index=3) -> (element=w417:cluster{string[]})
                n248 = call <vilib>:"NT Read String.vi"("name"=w419) -> ("value"=w418:string)  [unwired: 8 in, 2 out]
                n249 = Unbundle(w417) -> (w413:string[])
                n250 = Match First String(2:w413, 3:w418) -> (0:w414:i32)  [unwired: 1 out]
                n251 = property on="Test Ring" class="Ring (strict)"("Value"=w414, "Strings []"=w413) -> ()  [unwired: 2 in, 2 out]
                n252 = property on="Test Ring" class="Ring (strict)"("Visible"=TRUE) -> ()  [unwired: 2 in, 2 out]
                n253 = property on="Test Slider" class="Slide (strict)"("Visible"=FALSE) -> ()  [unwired: 2 in, 2 out]
              }
              frame "Color Enable  **" {
                n254 = Index Array(array=w425, index=4) -> (element=w426:cluster{string[]})
                n255 = call <vilib>:"NT Read String.vi"("name"=w428) -> ("value"=w427:string)  [unwired: 8 in, 2 out]
                n256 = Unbundle(w426) -> (w422:string[])
                n257 = Match First String(2:w422, 3:w427) -> (0:w423:i32)  [unwired: 1 out]
                n258 = property on="Test Ring" class="Ring (strict)"("Value"=w423, "Strings []"=w422) -> ()  [unwired: 2 in, 2 out]
                n259 = property on="Test Ring" class="Ring (strict)"("Visible"=TRUE) -> ()  [unwired: 2 in, 2 out]
                n260 = property on="Test Slider" class="Slide (strict)"("Visible"=FALSE) -> ()  [unwired: 2 in, 2 out]
              }
              frame Default {
                n261 = property on="Test Ring" class="Ring (strict)"("Visible"=FALSE) -> ()  [unwired: 2 in, 2 out]
                n262 = property on="Test Slider" class="Slide (strict)"("Visible"=FALSE) -> ()  [unwired: 2 in, 2 out]
              }
              frame "Brightness  **", "Color Level  **", "Compression  **", "FPS  **", "Sharpness  **" {
                n263 = call <vilib>:"NT Read Number.vi"("name"=w434) -> ("value"=w433:dbl)  [unwired: 8 in, 2 out]
                n264 = local write "Test Slider"(w433) -> ()
                n265 = property on="Test Slider" class="Slide (strict)"("Visible"=TRUE, "Scale.Maximum"=100.0 ("Scale.Range:Maximum")) -> ()  [unwired: 2 in, 2 out]
                n266 = property on="Test Ring" class="Ring (strict)"("Visible"=FALSE) -> ()  [unwired: 2 in, 2 out]
              }
            }
          }
        }
        n267 = property on="Progress" class="Clust (strict)"("Visible"=FALSE) -> ()  [unwired: 2 in, 2 out]
      }
      event "Test Name": Mouse Enter {
        # "Populate the ring with the list of tests"
        n268 = event-data() -> ()  [unwired: 1 in, 1 out]
        n269 = call <vilib>:"NT Read String Array.vi"("name"="TestMode/TestList" ("Name")) -> ("value"=w441:string[])  [unwired: 8 in, 2 out]
        n270 = Build Array (concatenate)("Select the test to run...", w441) -> (w440:string[])
        n271 = property on="Test Name" class="Ring (strict)"("Strings []"=w440) -> ()  [unwired: 2 in, 2 out]
      }
      event "Test Name": Value Change {
        w442 = FALSE ("Visible")
        # "Tell the robot the test name to run"
        n272 = event-data() -> ("NewVal"=w446:u16)  [unwired: 1 in]
        n273 = property on="Test Name" class="Ring (strict)"() -> ("Strings []"=w447:string[])  [unwired: 2 in, 2 out]
        n274 = local write "Progress"(T6 {"Test Progress"=0, "Test Progress Text"=""} ("Progress")) -> ()
        n275 = Index Array(array=w447, index=w446) -> (element=w445:string)
        n276 = call <vilib>:"NT Write String.vi"("value"=w445, "name"="TestMode/TestName" ("Name")) -> ()  [unwired: 9 in, 1 out]
        n277 = property on="Progress" class="Clust (strict)"("Visible"=TRUE) -> ()  [unwired: 2 in, 2 out]
        n278 = property on="Motor" class="Clust (strict)"("Visible"=w442) -> ()  [unwired: 2 in, 2 out]
        n279 = property on="Test Slider" class="Slide (strict)"("Visible"=w442) -> ()  [unwired: 2 in, 2 out]
        n280 = property on="On/Off" class="Bool (strict)"("Visible"=w442) -> ()  [unwired: 2 in, 2 out]
        n281 = property on="Rev/Fwd" class="Clust (strict)"("Visible"=w442) -> ()  [unwired: 2 in, 2 out]
        n282 = property on="Test Ring" class="Ring (strict)"("Visible"=w442) -> ()  [unwired: 2 in, 2 out]
      }
      event "Select Auto": Mouse Enter {
        # "Populate the combo box with the list of autonomous options"
        n283 = event-data() -> ()  [unwired: 1 in, 1 out]
        n284 = call <vilib>:"NT Read String Array.vi"("name"="Auto List" ("Name")) -> ("value"=w449:string[])  [unwired: 8 in, 2 out]
        n285 = property on="Select Auto" class="CmbBox"("Strings[]"=w449) -> ()  [unwired: 2 in, 2 out]
      }
      event "Select Auto": Value Change {
        # "User modified the Auto Selection. Write to NT variable so robot knows."
        n286 = event-data() -> ("NewVal"=w451:string)  [unwired: 1 in]
        n287 = call <vilib>:"NT Write String.vi"("value"=w451, "name"="Auto Selector" ("Name")) -> ()  [unwired: 9 in, 1 out]
      }
      event "CheckList": Double Click {
        # "Shift clears all"
        # "Update symbols on the listbox"
        n288 = event-data() -> ("PlatMods.Shift"=w453:bool, "Row"=w455:i32)  [unwired: 1 in]
        n289 = case shown="True" w453 {
          tunnel: w455 -> [w459 _]
          tunnel: 1 -> [w458 _]
          frame False {
            n290 = property on="CheckList" class="LstBox (strict)"() -> ("Item Symbols"=w457:i32[])  [unwired: 2 in, 2 out]
            n291 = Replace Array Subset(array=w457, new element=w458, index=w459) -> (w456:i32[])
            n292 = property on="CheckList" class="LstBox (strict)"("Item Symbols"=w456) -> ()  [unwired: 2 in, 2 out]
          }
          frame True {
            w460 = 0 ("Top Row")
            n293 = property on="CheckList" class="LstBox (strict)"() -> ("Number of Rows"=w462:u32)  [unwired: 2 in, 2 out]
            n294 = Initialize Array(0, w462) -> (w461:i32[])
            n295 = property on="CheckList" class="LstBox (strict)"("Top Row"=w460, "Value"=w460, "Item Symbols"=w461) -> ()  [unwired: 2 in, 2 out]
          }
        }
      }
      event "CheckList": Key Down {
        # "Update symbols on the listbox\nLeft and right keys check and uncheck"
        n296 = event-data() -> ("VKey"=w465:T24)  [unwired: 1 in]
        n297 = case shown="\"Left\", \"Right\"" w465 {
          selector: w465 -> [w470 _]
          tunnel: eventvkey."Left" ("VKey") -> [w468 _]
          frame "Left", "Right" {
            n298 = Equal?(x=w468, y=w470) -> (x = y?=w469:bool)
            n299 = Select(t=0, s=w469, f=1) -> (s? t:f=w471:i32)
            n300 = property on="CheckList" class="LstBox (strict)"() -> ("Item Symbols"=w474:i32[])  [unwired: 2 in, 2 out]
            n301 = Replace Array Subset(array=w474, new element=w471, index="CheckList") -> (w473:i32[])
            n302 = property on="CheckList" class="LstBox (strict)"("Item Symbols"=w473) -> ()  [unwired: 2 in, 2 out]
          }
          frame Default {
          }
        }
      }
      event "Motor.Enable": Value Change {
        # "When the test mode otor enable helper is set, update that\ntree row item's value"
        n303 = event-data() -> ("NewVal"=w479:bool)  [unwired: 1 in]
        n304 = Unbundle("Motor") -> ("Value"=w478:dbl)  [unwired: 1 out]
        n305 = Select(t=w478, s=w479, f=0.0) -> (s? t:f=w476:dbl)
        n306 = call <vilib>:"NT Write Number.vi"("value"=w476, "name"=w475) -> ()  [unwired: 9 in, 1 out]
      }
      event "Test Slider": Value Change {
        # "When the test mode slider helper is set, update that\ntree row item's value"
        n307 = event-data() -> ("NewVal"=w481:dbl)  [unwired: 1 in]
        n308 = call <vilib>:"NT Write Number.vi"("value"=w481, "name"=w482) -> ()  [unwired: 9 in, 1 out]
      }
      event "On/Off": Value Change {
        # "When the test mode on/off helper value is set, update that\ntree row item's value"
        n309 = event-data() -> ("NewVal"=w485:bool)  [unwired: 1 in]
        n310 = Boolean To (0,1)(Boolean=w485) -> (0, 1=w484:i16)
        n311 = call <vilib>:"NT Write Number.vi"("value"=w484, "name"=w483) -> ()  [unwired: 9 in, 1 out]
      }
      event "Rev/Fwd": Value Change {
        # "When the test mode helper value for relays is set, update that\ntree row item's value"
        n312 = event-data() -> ("NewVal.Forward"=w492:bool, "NewVal.Reverse"=w491:bool)  [unwired: 1 in]
        n313 = Boolean To (0,1)(Boolean=w492) -> (0, 1=w488:i16)
        n314 = Boolean To (0,1)(Boolean=w491) -> (0, 1=w490:i16)
        n315 = Negate(x=w490) -> (-x=w489:i16)
        n316 = Add(x=w488, y=w489) -> (x+y=w487:i16)
        n317 = call <vilib>:"NT Write Number.vi"("value"=w487, "name"=w486) -> ()  [unwired: 9 in, 1 out]
      }
      event "Test Ring": Value Change {
        # "When a test mode helper value is selected from the ring,\nset the tree item's variable to the string value"
        n318 = event-data() -> ("NewVal"=w495:u16)  [unwired: 1 in]
        n319 = property on="Test Ring" class="Ring (strict)"() -> ("Strings []"=w496:string[])  [unwired: 2 in, 2 out]
        n320 = Index Array(array=w496, index=w495) -> (element=w494:string)
        n321 = call <vilib>:"NT Write String.vi"("value"=w494, "name"=w493) -> ()  [unwired: 9 in, 1 out]
      }
      event "Rec Mode": Value Change {
        # "Update globals for recording mode and path to read log from.\nClear when logging and let NetworkTables set path for vision to\nuse."
        n322 = event-data() -> ("NewVal"=w505:enum32{"Stop", "Record", "Playback"})  [unwired: 1 in]
        n323 = global write "WPI_DashboardLogging Global.vi" "Logging Filename"(path "") -> ()
        n324 = global write "WPI_DashboardLogging Global.vi" "Recording"(w505) -> ()
        n325 = case shown="\"Playback\"" w505 {
          tunnel: w504 -> [_ w507 w515]
          tunnel: [_ _ w514] -> w502
          tunnel: [_ _ w513] -> _
          tunnel: w500 -> [_ _ w511]
          tunnel: cluster{i32, i32} {-250, 170} -> [_ _ w510]
          tunnel: [_ _ T25 {"Image Size"=TRUE, "Image Type"=TRUE, "Pixel Value"=TRUE, "ROI Information"=TRUE, "Zoom Factor"=FALSE} ("Image Information Shown:All Elements")] -> w497
          tunnel: [_ _ TRUE ("Zoom Factor")] -> w498
          frame Default {
          }
          frame "Stop", "Record" {
            # "Place Window too"
            n326 = invoke class="VI" method="FP.Close"(reference=w507) -> (reference out=w506:refnum<vi>)  [unwired: 2 in, 2 out]
            n327 = invoke class="VI" method="Abort VI"(reference=w506) -> ()  [unwired: 2 in, 3 out]
          }
          frame "Playback" {
            n328 = call "Open Playback Panel.vi"("Offset"=w510, "DB VI Ref"=w511, "Playback in"=w515) -> ("Playback out"=w512:refnum<vi>)  [unwired: 8 in]
            n329 = register-events(w512) -> (reference out=w514:refnum<event-registration>, error out=w513:errorcluster)  [unwired: 2 in]
          }
        }
        n330 = property on="Camera Image Right" class="ImageControl"("Image Information Shown"=w497, "Image Information Visible"=w498) -> ()  [unwired: 2 in, 2 out]
        n331 = property on="Camera Image" class="ImageControl"("Image Information Shown"=w497, "Image Information Visible"=w498) -> ()  [unwired: 2 in, 2 out]
        n332 = call <vilib>:"WPI_DashboardNT Log FieldName Cache.vi"("Operation"=enum16{"Lookup/Add", "Index", "Clear"}."Clear") -> ()  [unwired: 8 in, 3 out]
      }
      event Panel Close {
        w516 = enum32{"Stop", "Record", "Playback"}."Stop" ("Rec Mode")
        # "Playback window has been closed, abort"
        n333 = event-data() -> ()  [unwired: 1 in, 4 out]
        n334 = local write "Rec Mode"(w516) -> ()
        n335 = global write "WPI_DashboardLogging Global.vi" "Recording"(w516) -> ()
      }
      event Panel Close {
        # "Abort playback window and ourself"
        n336 = event-data() -> ()  [unwired: 1 in, 4 out]
        n337 = invoke class="VI" method="FP.Close"(reference=w519) -> (reference out=w518:refnum<vi>)  [unwired: 2 in, 2 out]
        n338 = invoke class="VI" method="Abort VI"(reference=w518) -> (error out=w517:errorcluster)  [unwired: 2 in, 2 out]
        n339 = invoke class="VI" method="Abort VI"(error in=w517) -> ()  [unwired: 2 in, 3 out]
      }
      event "Tree": Double Click {
        n340 = event-data() -> ("PlatMods"=w525:T27, "Tag"=w522:string)  [unwired: 1 in]
        n341 = Unbundle(w525) -> ("Shift"=w524:bool)  [unwired: 4 out]
        n342 = String Subset(string=w522, length (rest)=1 ("length (rest)")) -> (substring=w521:string)  [unwired: 1 in]
        n343 = Not(x=w524) -> (.not. x?=w523:bool)
        n344 = case shown="\"/\"" w521 {
          tunnel: w522 -> [_ w527]
          tunnel: w523 -> [_ w526]
          frame Default {
          }
          frame "/" {
            n345 = call <vilib>:"NT Update Persistence.vi"("Persistence"=w526, "Name"=w527) -> ()  [unwired: 9 in, 1 out]
          }
        }
      }
    }
  }
  n346 = while {
    tunnel: w96 -> [w529]
    i -> [w532]
    stop <- FALSE stop-if-true
    n347 = Wait (ms)(milliseconds to wait=u32 100) -> ()  [unwired: 1 out]
    n348 = case shown="\"Playback\"" "Rec Mode" {
      tunnel: w532 -> [_ _ w547]
      tunnel: [u32 2829099 ("Base Color") u32 11141120 ("Target Color") w536] -> w528
      frame "Stop", Default {
        # "Reset the color, extra updates don't cost much"
      }
      frame "Record" {
      }
      frame "Playback" {
        # "Playback"
        n349 = Quotient & Remainder(x=w547, y=u32 50 ("milliseconds to wait")) -> (x-y*floor(x/y)=w543:u32)  [unwired: 1 out]
        n350 = Divide(x=w543, y=u32 50 ("milliseconds to wait")) -> (x/y=w540:dbl)
        n351 = Multiply(x=6.283185307179586, y=w540) -> (x*y=w545:dbl)
        n352 = Sine(x=w545) -> (sin(x)=w544:dbl)
        n353 = Absolute Value(x=w544) -> (abs(x)=w537:dbl)
        n354 = call "Interpolate RGB Color.vi"("Proportion"=w537, "Target Color"=u32 30976, "Base Color"=u32 2829099) -> ("Result Color"=w536:u32)  [unwired: 8 in]
      }
    }
    n355 = property class="Pane"(reference=w529, "PaneColor"=w528) -> ()  [unwired: 1 in, 2 out]
  }
  n356 = local write "Dashboard Tab"(T2."Drive" ("Dashboard Tab")) -> ()
  n357 = property on="On/Off" class="Bool (strict)"("Visible"=w68) -> ()  [unwired: 2 in, 2 out]
  n358 = property on="Motor" class="Clust (strict)"("Visible"=w68) -> ()  [unwired: 2 in, 2 out]
  n359 = property on="Progress" class="Clust (strict)"("Visible"=w68) -> ()  [unwired: 2 in, 2 out]
  n360 = property on="Test Ring" class="Ring (strict)"("Visible"=w68) -> ()  [unwired: 2 in, 2 out]
  n361 = property on="Rev/Fwd" class="Clust (strict)"("Visible"=w68) -> ()  [unwired: 2 in, 2 out]
  n362 = while {
    tunnel: u16 1741 ("timeout ms (25000)") -> [w549]
    stop <- FALSE stop-if-true
    n363 = TCP Create Listener(10:w549) -> (0:w548:errorcluster, 3:w550:refnum<k5>)  [unwired: 4 in, 1 out]
    n364 = case shown="No Error" w548 {
      selector: w548 -> [w552 _]
      tunnel: w550 -> [w553 _]
      frame No Error {
        n365 = while {
          tunnel: w553 -> [w556]
          tunnel: w552 -> [w555]
          stop <- FALSE stop-if-true
          n366 = TCP Wait On Listener(8:w555, 11:w556) -> (0:w557:errorcluster, 4:w558:refnum<k5>)  [unwired: 2 in, 3 out]
          n367 = local write "TCP"(w558) -> ()
          n368 = case shown="Error" w557 {
            frame No Error {
            }
            frame Error {
              n369 = Wait (ms)(milliseconds to wait=u32 1000) -> ()  [unwired: 1 out]
            }
          }
        }
      }
      frame Error {
        n370 = Wait (ms)(milliseconds to wait=u32 1000) -> ()  [unwired: 1 out]
      }
    }
  }
  n371 = global write "WPI_DashboardLogging Global.vi" "Recording"(w91) -> ()
  n372 = local write "Rec Mode"(w91) -> ()
  n373 = call <vilib>:"NT Write String.vi"("value"="Select Auto", "name"="Auto Selector" ("Name")) -> ()  [unwired: 9 in, 1 out]
  n374 = control-ref of="Field"() -> (w4:refnum<vi>)
  n375 = property on="Property Node" class="XYGraph (strict)"(reference=w4) -> ("Width"=w6:u32, "Height"=w7:u32)  [unwired: 1 in, 2 out]
  n376 = Divide(x=26.0, y=649.0) -> (x/y=w22:dbl)
  n377 = Divide(x=24.0, y=319.0) -> (x/y=w25:dbl)
  n378 = Multiply(x=w22, y=2.0) -> (x*y=w21:dbl)
  n379 = Multiply(x=w25, y=2.0) -> (x*y=w20:dbl)
  n380 = call "IMAQ Create"("Image Name"="Field image", "Image Type"=w40) -> ("New Image"=w3:T5)  [unwired: 3 in, 1 out]
  n381 = call <vilib>:"Picture to Pixmap.vi"("picture"=picture bytes[1973190] ("new picture")) -> ("image data"=w2:T28)  [unwired: 9 in, 1 out]
  n382 = Divide(x=26.0, y=319.0) -> (x/y=w15:dbl)
  n383 = Divide(x=20.0, y=649.0) -> (x/y=w14:dbl)
  n384 = Increment(x=w21) -> (x+1=w19:dbl)
  n385 = Increment(x=w20) -> (x+1=w18:dbl)
  n386 = Negate(x=w15) -> (-x=w13:dbl)
  n387 = Increment(x=w15) -> (x+1=w9:dbl)
  n388 = Negate(x=w14) -> (-x=w12:dbl)
  n389 = Increment(x=w14) -> (x+1=w8:dbl)
  n390 = call "Convert LabVIEW Image Data To IMAQ.vi"("Image Data"=w2, "Image In"=w3) -> ("Image Out"=w1:T5)  [unwired: 8 in, 1 out]
  n391 = Multiply(x=w6, y=w19) -> (x*y=w17:dbl)
  n392 = Multiply(x=w7, y=w18) -> (x*y=w16:dbl)
  n393 = Multiply(x=w9, y=w7) -> (x*y=w11:dbl)
  n394 = Multiply(x=w8, y=w6) -> (x*y=w10:dbl)
  n395 = call "IMAQ Resample"("X Resolution"=w17, "Y Resolution"=w16, "Image Src"=w1) -> ("Image Dst Out"=w39:T5)  [unwired: 7 in, 1 out]
  n396 = Multiply(x=w13, y=w11) -> (x*y=w31:dbl)
  n397 = Multiply(x=w12, y=w10) -> (x*y=w32:dbl)
  n398 = call "IMAQ ColorImageToArray"("Image"=w39) -> ("Image Pixels (U32)"=w38:u32[][])  [unwired: 3 in, 2 out]
  n399 = Bundle(cluster=cluster{"x":i16, "y":i16} {"x"=0, "y"=0} ("top left point(0, 0)"), "x"=w31, "y"=w32) -> (w30:cluster{"x":i16, "y":i16})
  n400 = call-poly <vilib>:"Draw Unflattened Pixmap.vi"("top left point(0, 0)"=w30, "data (RGB format)"=w38) -> ("new picture"=w5:picture)  [unwired: 7 in]
  n401 = property class="XYGraph (strict)"(reference=w4, "PlotImages.Back"=w5) -> ()  [unwired: 1 in, 2 out]
